vi "General-GenerateSineWaveForm.vi"(0 "tiempo (s)":sgl, 1 "#samples":u32, 2 "Amplitud":dbl, 3 "frecuencia":dbl, 4 "Fs (S/s)":dbl, 5 "df":dbl[](array[numeric])) -> (7 "Waveform":waveform(dbl)(graph))   [LabVIEW 2010]
panel:
  out "Waveform Graph":dbl[](graph)
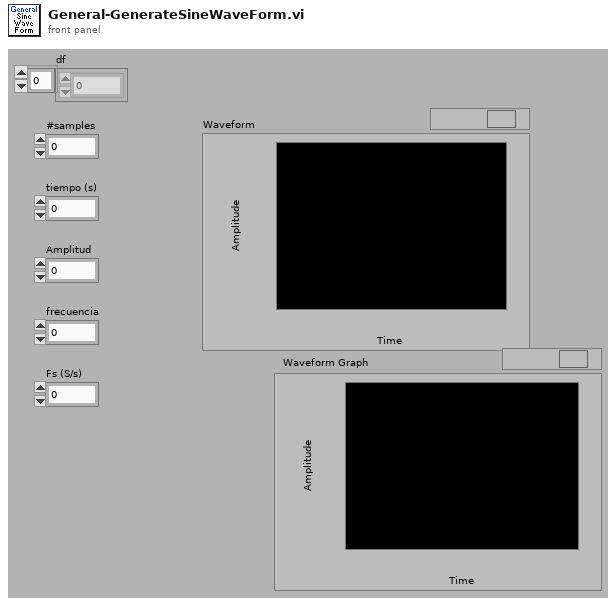
[diagram p1: front panel]
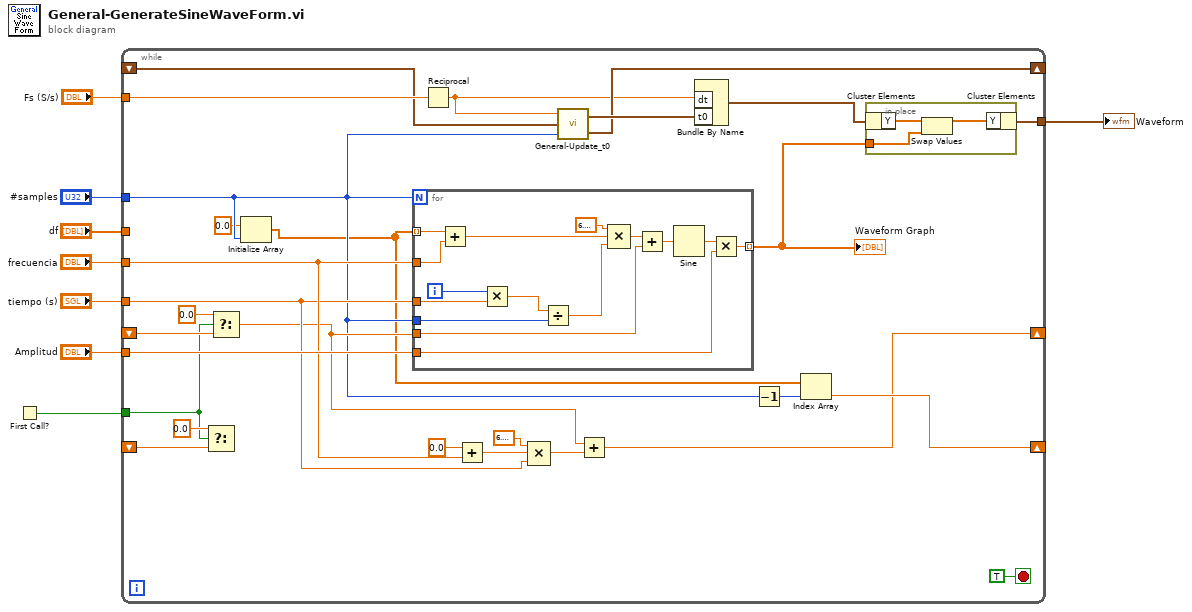
[diagram p0: block diagram]
diagram:
  n1 = First Call?() -> (First Call?: T/F=w1:bool)
  n2 = while {
    tunnel: "#samples" -> [w11]
    tunnel: "tiempo (s)" -> [w24]
    tunnel: "frecuencia" -> [w27]
    tunnel: "Amplitud" -> [w35]
    shift-right: [w22] -> _
    shift-left: _ -> [w19]
    tunnel: "Fs (S/s)" -> [w34]
    shift-right: [w30] -> _
    shift-left: _ -> [w32]
    tunnel: [w20] -> w8
    tunnel: "df" -> [_]
    shift-right: [w28] -> _
    shift-left: _ -> [w15]
    tunnel: w1 -> [w14]
    stop <- TRUE ("Boolean") stop-if-true
    n3 = Select(t=0.0, s=w14, f=w15) -> ()  [unwired: 1 out]
    n4 = Select(t=0.0, s=w14, f=w19) -> (s? t:f=w18:dbl)
    n5 = Initialize Array(0.0 ("element"), w11) -> (w10:dbl[])
    n6 = for {
      N: w11 -> [_]
      tunnel: w24 -> [w53]
      tunnel: w27 -> [w44]
      tunnel: w18 -> [w50]
      tunnel: w35 -> [w48]
      tunnel: w11 -> [w42]
      tunnel: w10 -> [w41] mode=indexing
      tunnel: [w40] -> w12 mode=indexing
      i -> [w54]
      n7 = Add(x=w41, y=w44) -> (x+y=w43:dbl)
      n8 = Multiply(x=w54, y=w53) -> (x*y=w52:sgl)
      n9 = Divide(x=w52, y=w42) -> (x/y=w46:sgl)
      n10 = Compound Arithmetic op=MULTIPLY(6.283185307179586, w43, w46) -> (w45:dbl)
      n11 = Add(x=w45, y=w50) -> (x+y=w51:dbl)
      n12 = Sine(x=w51) -> (sin(x)=w49:dbl)
      n13 = Multiply(x=w49, y=w48) -> (x*y=w40:dbl)
    }
    "Waveform Graph" <- w12
    n14 = Reciprocal(x=w34) -> (1/x=w21:dbl)
    n15 = Add(x=0.0, y=w27) -> (x+y=w25:dbl)
    n16 = Compound Arithmetic op=MULTIPLY(6.283185307179586, w25, w24) -> (w23:dbl)
    n17 = call "General-Update_t0.vi"("#samples"=w11, "t0 IN"=w32, "dt"=w21) -> ("tf new"=w30:timestamp, "t0 OUT"=w31:timestamp)
    n18 = Add(x=w18, y=w23) -> (x+y=w22:dbl)
    n19 = Bundle By Name("dt"=w21, "t0"=w31) -> (w33:waveform(dbl))  [unwired: 1 in]
    n20 = Decrement(x=w11) -> (x-1=w29:u32)
    n21 = Index Array(array=w10, index=w29) -> (element=w28:dbl)
    n22 = in-place {
      in-place-border: w12 -> [w37]
      n23 = in-place-cluster #1(w33) -> ("Y"=w39:dbl[])
      n24 = Swap Values(12:w39, 14:w37) -> (1:w38:dbl[])  [unwired: 1 in, 1 out]
      n25 = in-place-cluster #1("Y"=w38) -> (w20:waveform(dbl))
    }
  }
  "Waveform" <- w8
